vi "TS Readout.vi"() -> ()   [LabVIEW 2023]
uses:
  <vilib>/FPGAPlugInAG/NI 9147/niLvFpga_Open_NI 9147.vi
  <vilib>/rvi/interface/common/dynamic/niFpgaDynamicAddResources.vi
  <vilib>/Utility/error.llb/Error Cluster From Error Code.vi
  <vilib>/rvi/errors/niLvFpgaAdjustHostInterfaceError.vi
  <vilib>/RVI Host/nirviSupport.llb/nirviErrorClusterFromErrorCode.vi
  <vilib>/FPGAPlugInAG/Dynamic/niLvFpga_Close_Dynamic.vi
  <vilib>/rvi/interface/nirviOpenFPGA/nirviOpenFPGA.xnode
  FPGA Bitfiles/ThermalScanner_FPGA.lvbitx
  FPGA.vi
  <vilib>/rvi/interface/nirviReadWriteControl/nirviReadWriteControl.xnode
  <vilib>/rvi/interface/nirviMethod/nirviMethod.xnode
  <vilib>/rvi/interface/nirviCloseFPGA/nirviCloseFPGA.xnode
  NiFpgaLv.dll
  <vilib>/rvi/interface/Simulation/niFpgaSimulationCallBeginRW.vi
  <vilib>/FPGAPlugInAG/Dynamic/niLvFpga_ReadFifo_Dynamic.vi
  <vilib>/rvi/errors/niLvFpgaMergeErrorWithErrorCode.vi
  <vilib>/rvi/interface/nirviMethod/StockFPGA_InlinedMethodWaitForSingleIRQ.vi
  <vilib>/FPGAPlugInAG/Dynamic/niLvFpga_WaitOnIrq_Dynamic.vi
  <vilib>/FPGAPlugInAG/Dynamic/niLvFpga_AcknowledgeIrq_Dynamic.vi
panel:
  out "Open":bool[](array[boolean])
  out "Out Of Range":bool[](array[boolean])
  out "NIST Calibrated (degC)":dbl[](array[numeric]) format="%.4f"
  out "Loop Count":i32
  out "Busy LED":bool
  out "date/time string":string
  out "Raw (V)":fxp<+/-,24,-2>[](array[numeric]) format="%#_12g"
  in  "Capture":bool
  in  "Data file":path
  out "FIFO Size":u32
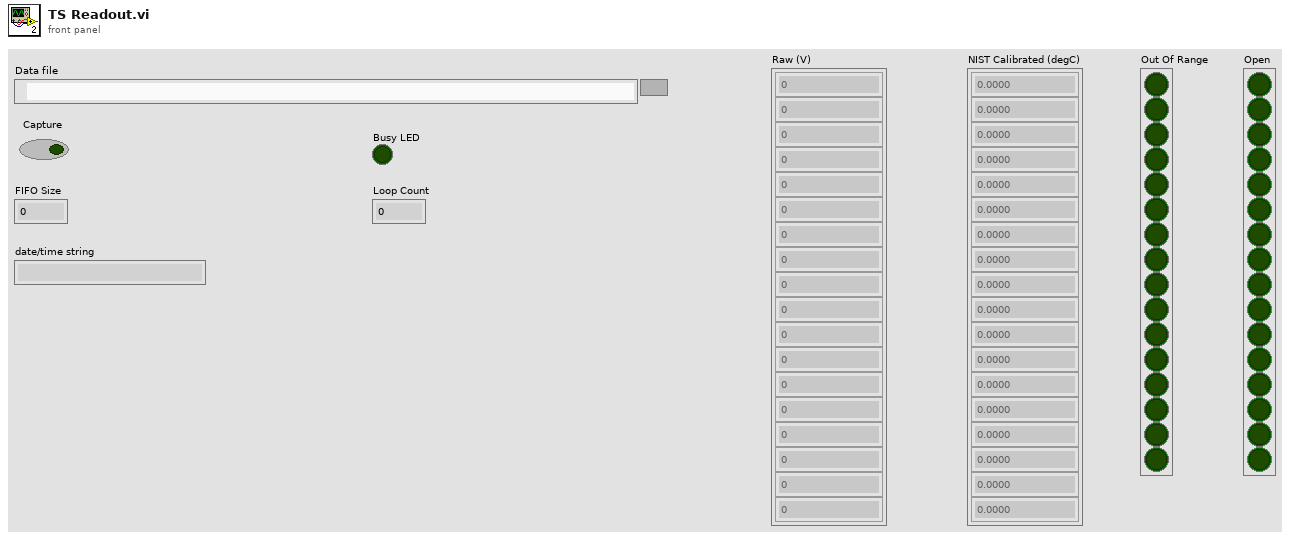
[diagram p1: front panel]
types:
  T1 = enum16{"open", "replace", "create", "open or create", "replace or create", "replace or create with confirmation"}
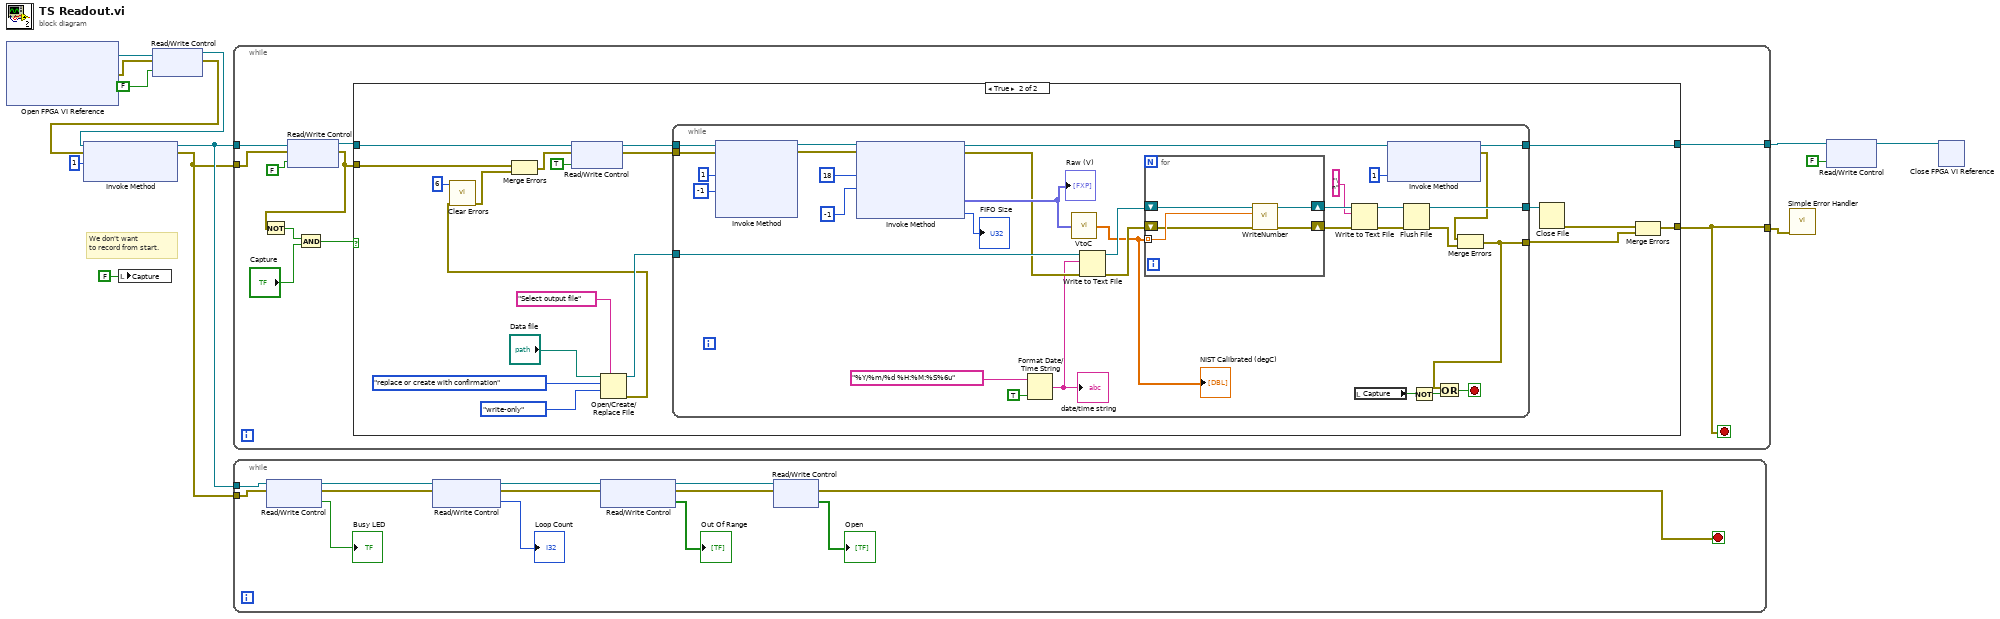
[diagram p0: block diagram]
diagram:
  # "We don't want\nto record from start."
  n1 = xnode "Open FPGA VI Reference"() -> ("FPGA VI Reference Out"=w4:refnum<k20>, "error out"=w3:errorcluster)  [unwired: 2 in]
  n2 = local write "Capture"(FALSE ("Capture")) -> ()
  n3 = xnode "Read/Write Control"("FPGA VI Reference In"=w4, "error in"=w3, "Capture"=FALSE) -> ("FPGA VI Reference Out"=w1:refnum<k20>, "error out"=w2:errorcluster)
  n4 = xnode "Invoke Method"("FPGA VI Reference In"=w1, "error in"=w2, "IRQ Number(s)"=1) -> ("FPGA VI Reference Out"=w6:refnum<k20>, "error out"=w5:errorcluster)
  n5 = while {
    tunnel: w6 -> [w17]
    tunnel: w5 -> [w15]
    tunnel: [w20] -> w13
    tunnel: [w19] -> w11
    stop <- w20 stop-if-true
    n6 = xnode "Read/Write Control"("FPGA VI Reference In"=w17, "error in"=w15, "Capture"=FALSE) -> ("FPGA VI Reference Out"=w16:refnum<k20>, "error out"=w14:errorcluster)
    n7 = Not(x=w14) -> (.not. x?=w21:bool)
    n8 = And(x=w21, y="Capture") -> (x .and. y?=w22:bool)
    n9 = case shown="True" w22 {
      tunnel: w16 -> [w24 w37]
      tunnel: w14 -> [w25 w36]
      tunnel: [w25 w33] -> w20
      tunnel: [w24 w30] -> w19
      frame False {
      }
      frame True {
        n10 = Open/Create/Replace File(file path (use dialog)="Data file", prompt="Select output file", operation (0:open)=T1."replace or create with confirmation", access (0:read/write)=enum16{"read/write", "read-only", "write-only"}."write-only") -> (refnum out=w34:refnum<file>, error out=w27:errorcluster)  [unwired: 2 in, 1 out]
        n11 = call <vilib>:"Clear Errors.vi"("error in (no error)"=w27, "specific error code to clear (0: all)"=6) -> ("error out"=w26:errorcluster)  [unwired: 4 in, 1 out]
        n12 = Merge Errors(w36, w26) -> (w35:errorcluster)
        n13 = xnode "Read/Write Control"("FPGA VI Reference In"=w37, "error in"=w35, "Capture"=TRUE) -> ("FPGA VI Reference Out"=w40:refnum<k20>, "error out"=w38:errorcluster)
        n14 = while {
          tunnel: w40 -> [w56]
          tunnel: w38 -> [w55]
          tunnel: [w49] -> w30
          tunnel: w34 -> [w71]
          tunnel: [w46] -> w31
          tunnel: [w65] -> w29
          stop <- w70 stop-if-true
          n15 = xnode "Invoke Method"("FPGA VI Reference In"=w56, "error in"=w55, "IRQ Number(s)"=1, "Timeout (ms)"=-1) -> ("FPGA VI Reference Out"=w53:refnum<k20>, "error out"=w54:errorcluster)  [unwired: 2 out]
          n16 = xnode "Invoke Method"("FPGA VI Reference In"=w53, "error in"=w54, "Number of Elements"=u32 18, "Timeout (ms)"=-1) -> ("FPGA VI Reference Out"=w50:refnum<k20>, "error out"=w69:errorcluster, "Data"=w74:fxp<+/-,24,-2>[], "Elements Remaining"=→"FIFO Size":u32)
          "Raw (V)" <- w74
          n17 = Format Date/Time String(time format string (%c)="%Y/%m/%d %H:%M:%S%6u", UTC format=TRUE) -> (date/time string=w66:string)  [unwired: 1 in]
          "date/time string" <- w66
          n18 = call "VtoC.vi"("Input"=w74) -> ("Output"=w57:dbl[])
          "NIST Calibrated (degC)" <- w57
          n19 = Write to Text File(file (use dialog)=w71, text=w66, error in=w69) -> (refnum out=w59:refnum<file>, error out=w58:errorcluster)  [unwired: 1 in, 1 out]
          n20 = for {
            shift-right: [w81] -> w64
            shift-left: w59 -> [w82]
            tunnel: w57 -> [w80] mode=indexing
            shift-right: [w79] -> w63
            shift-left: w58 -> [w78]
            n21 = call "WriteNumber.vi"("error in (no error)"=w78, "Numeric"=w80, "Byte Stream File in"=w82) -> ("error out"=w79:errorcluster, "Byte Stream File out"=w81:refnum<file>)  [unwired: 7 in]
          }
          n22 = Write to Text File(file (use dialog)=w64, text="\n", error in=w63) -> (refnum out=w60:refnum<file>, error out=w61:errorcluster)  [unwired: 1 in, 1 out]
          n23 = local read "Capture"() -> (w76:bool)
          n24 = xnode "Invoke Method"("FPGA VI Reference In"=w50, "IRQ Number(s)"=1) -> ("FPGA VI Reference Out"=w49:refnum<k20>, "error out"=w48:errorcluster)  [unwired: 1 in]
          n25 = Flush File(refnum=w60, error in=w61) -> (refnum out=w65:refnum<file>, error out=w47:errorcluster)
          n26 = Not(x=w76) -> (.not. x?=w68:bool)
          n27 = Merge Errors(w48, w47) -> (w46:errorcluster)
          n28 = Or(x=w46, y=w68) -> (x .or. y?=w70:bool)
        }
        n29 = Close File(refnum=w29) -> (error out=w32:errorcluster)  [unwired: 1 in, 1 out]
        n30 = Merge Errors(w32, w31) -> (w33:errorcluster)
      }
    }
  }
  n31 = while {
    tunnel: w6 -> [w95]
    tunnel: w5 -> [w94]
    stop <- w85 stop-if-true
    n32 = xnode "Read/Write Control"("FPGA VI Reference In"=w95, "error in"=w94) -> ("FPGA VI Reference Out"=w92:refnum<k20>, "error out"=w91:errorcluster, "Busy LED"=→"Busy LED":bool)
    n33 = xnode "Read/Write Control"("FPGA VI Reference In"=w92, "error in"=w91) -> ("FPGA VI Reference Out"=w89:refnum<k20>, "error out"=w88:errorcluster, "Loop Count"=→"Loop Count":i32)
    n34 = xnode "Read/Write Control"("FPGA VI Reference In"=w89, "error in"=w88) -> ("FPGA VI Reference Out"=w87:refnum<k20>, "error out"=w86:errorcluster, "Out Of Range"=→"Out Of Range":bool[])
    n35 = xnode "Read/Write Control"("FPGA VI Reference In"=w87, "error in"=w86) -> ("error out"=w85:errorcluster, "Open"=→"Open":bool[])  [unwired: 1 out]
  }
  n36 = call <vilib>:"Simple Error Handler.vi"("error in (no error)"=w13) -> ()  [unwired: 4 in, 5 out]
  n37 = xnode "Read/Write Control"("FPGA VI Reference In"=w11, "Capture"=FALSE) -> ("FPGA VI Reference Out"=w10:refnum<k20>)  [unwired: 1 in, 1 out]
  n38 = xnode "Close FPGA VI Reference"("FPGA VI Reference In"=w10) -> ()  [unwired: 1 in, 1 out]
